vi "Initialize.vi"(6 "Actor Name":string, 7 "Host Name":string, 8 "error in (no error)":errorcluster, 11 "Message Broker Interface":refnum<class "Message Broker Interface.lvclass">) -> (0 "error out":errorcluster, 3 "Car Wash Station Sequencer out":refnum<class "Car Wash Station Sequencer.lvclass">)   [LabVIEW 2016, in "CLD Exam - Car Wash.lvlib" / "Car Wash Station Sequencer.lvclass"]
uses:
  Car Wash Station Sequencer.lvclass
  Mediator/Classes/Message Broker Interface/Message Broker Interface.lvclass
  Car Wash Station Sequencer.lvclass/Car Wash Station Sequencer.ctl
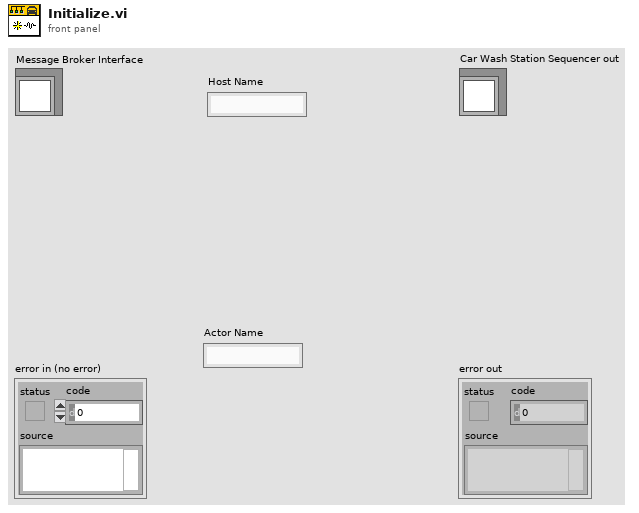
[diagram p1: front panel]
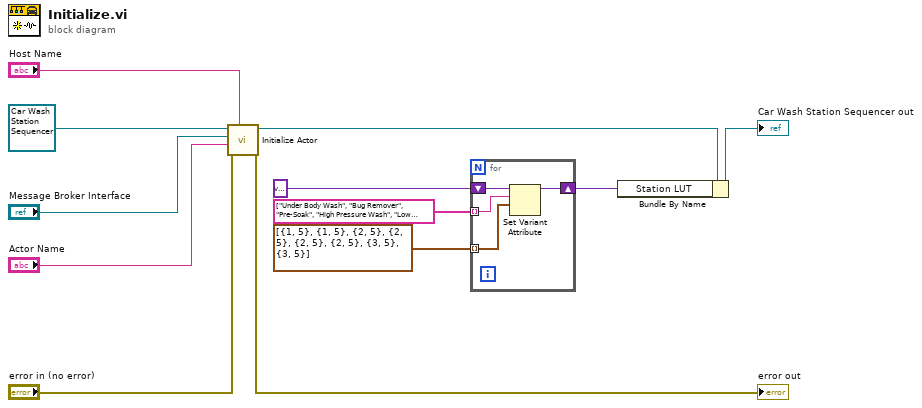
[diagram p0: block diagram]
diagram:
  n1 = call-dynamic "Initialize Actor.vi"("Host Name"="Host Name", "error in (no error)"="error in (no error)", "Actor Name"="Actor Name", "Message Broker Interface"="Message Broker Interface", "Car Wash Station Sequencer in"=refnum<class "Car Wash Station Sequencer.lvclass"> refnum) -> ("error out"=→"error out":errorcluster, "Car Wash Station Sequencer out"=w6:refnum<class "Car Wash Station Sequencer.lvclass">)  [unwired: 5 in]
  n2 = for {
    shift-right: [w15] -> w1
    shift-left: variant ("variant") -> [w16]
    tunnel: string[] ["Under Body Wash", "Bug Remover", "Pre-Soak", "High Pressure Wash", "Low Pressure Wax", "Spot Free Rinse", "Tire Shine Foam", "Air Dry"] -> [w14] mode=indexing
    tunnel: cluster{"Station":u8, "Step Time":u16}[] [{"Station"=1, "Step Time"=5}, {"Station"=1, "Step Time"=5}, {"Station"=2, "Step Time"=5}, {"Station"=2, "Step Time"=5}, {"Station"=2, "Step Time"=5}, {"Station"=2, "Step Time"=5}, {"Station"=3, "Step Time"=5}, {"Station"=3, "Step Time"=5}] -> [w13] mode=indexing
    n3 = Set Variant Attribute(Variant=w16, name=w14, value=w13) -> (Variant out=w15:variant)  [unwired: 1 in, 2 out]
  }
  n4 = Bundle By Name(cluster=w6, "Station LUT"=w1) -> (→"Car Wash Station Sequencer out":refnum<class "Car Wash Station Sequencer.lvclass">)
